vi "Cntrl_Ch_Status_low.vi"(1 "Mode":T1(ring), 2 "Channel names":string[](array[string])) -> (0 "Disabled Chs":string[](array[string]))   [LabVIEW 2020]
uses:
  Sub VIs/ADAM Controls/Channel_State.ctl
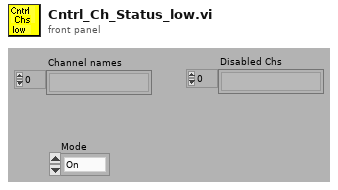
[diagram p1: front panel]
types:
  T1 = enum16{"On", "Off", "Always On", "Always Off", "Delete"}
  T2 = typedef "Channel_State.ctl" = enum16{"On", "Off", "Always On", "Always Off"}
  T3 = typedef "Ch_description_ADAM.ctl" = cluster{"Ch Name":string, "Type":T4, "Function":T5, "Ch State":T2, "Calibration type":T6, "A":dbl, "B":dbl, "C":dbl, "D":dbl, "Comments":string, "Address":T7, "String":string, "Duty":u16}
  T4 = typedef "Module_type_ADAM.ctl" = string
  T5 = typedef "Function_ADAM.ctl" = enum16{"Analogue Input", "Digital Input", "Event counter", "Event rate", "Analogue Output", "Digital Output", "Relay Output"}
  T6 = typedef "Calib_type_ADAM.ctl" = string
  T7 = typedef "Address.ctl" = cluster{"Main":i32, "Ch.":i32, "Sub":i32, "Port Name":string}
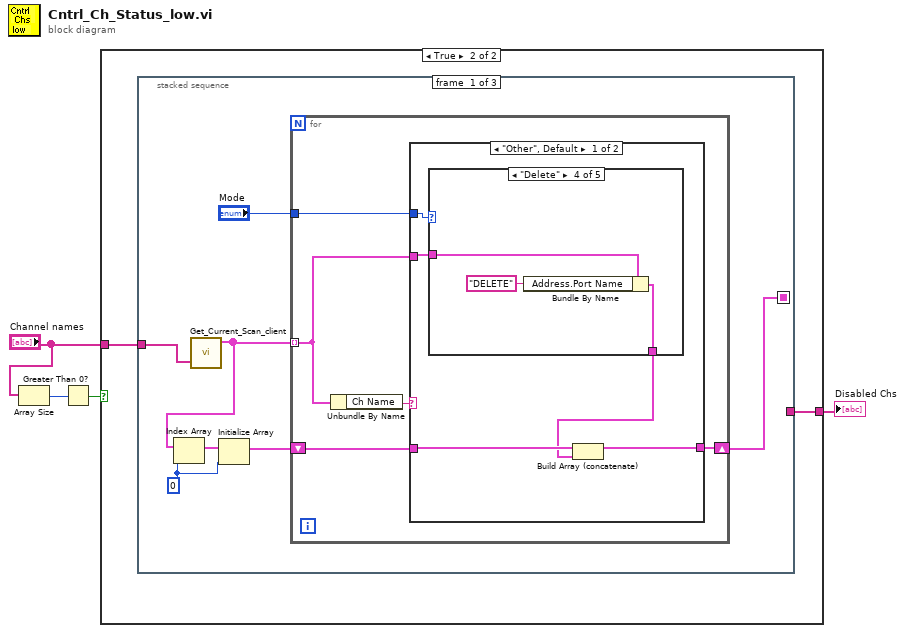
[diagram p0: block diagram]
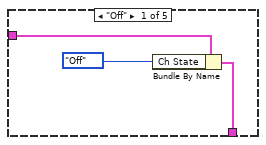
[diagram p3: hidden frame]
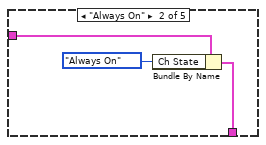
[diagram p4: hidden frame]
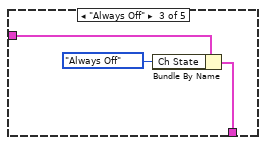
[diagram p5: hidden frame]
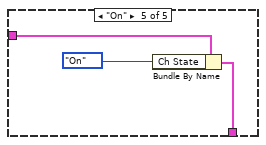
[diagram p6: hidden frame]
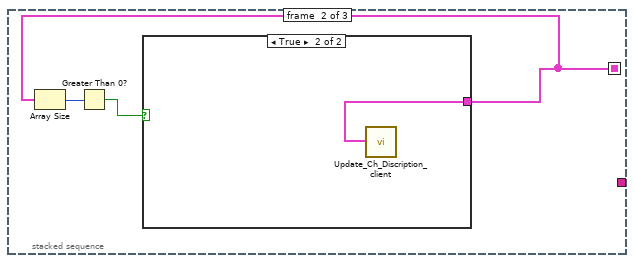
[diagram p8: hidden frame]
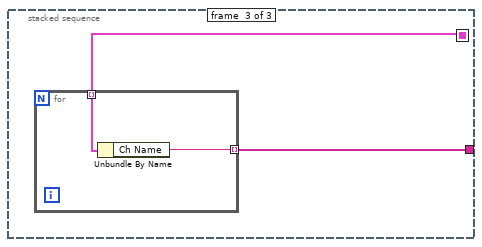
[diagram p10: hidden frame]
diagram:
  n1 = Array Size(array="Channel names") -> (size(s)=w4:i32)
  n2 = Greater Than 0?(x=w4) -> (x > 0?=w2:bool)
  n3 = case shown="True" w2 {
    tunnel: "Channel names" -> [w5 w7]
    tunnel: [w5 w6] -> w1
    frame False {
    }
    frame True {
      n4 = stacked-sequence {
        seq-local: [w9 _ _] -> [_ w41 w46]
        tunnel: w7 -> [w14 _ _]
        tunnel: [_ _ w45] -> w6
        frame #0 {
          w13 = 0 ("Index")
          n5 = call "Get_Current_Scan_client.vi"("multipleChannels"=w14) -> ("Ch Description Array"=w12:T3[])  [unwired: 2 in, 2 out]
          n6 = Index Array(array=w12, index=w13) -> (element=w11:T3)
          n7 = Initialize Array(w11, w13) -> (w10:T3[])
          n8 = for {
            tunnel: w12 -> [w16] mode=indexing
            shift-right: [w18] -> w9
            shift-left: w10 -> [w17]
            tunnel: "Mode" -> [w15]
            n9 = Unbundle By Name(w16) -> ("Ch Name"=w19:string)
            n10 = case shown="\"Other\", Default" w19 {
              tunnel: [w23 w40] -> w18
              tunnel: w17 -> [w24 w40]
              tunnel: w16 -> [w22 _]
              tunnel: w15 -> [w20 _]
              frame "Other", Default {
                n11 = case shown="\"Delete\"" w20 {
                  tunnel: w22 -> [w27 w30 w33 w36 w39]
                  tunnel: [w26 w29 w32 w35 w38] -> w21
                  frame "Off" {
                    n12 = Bundle By Name(cluster=w27, "Ch State"=Channel_State."Off" ("Channel State")) -> (w26:T3)
                  }
                  frame "Always On" {
                    n13 = Bundle By Name(cluster=w30, "Ch State"=Channel_State."Always On" ("Channel State")) -> (w29:T3)
                  }
                  frame "Always Off" {
                    n14 = Bundle By Name(cluster=w33, "Ch State"=Channel_State."Always Off" ("Channel State")) -> (w32:T3)
                  }
                  frame "Delete" {
                    n15 = Bundle By Name(cluster=w36, "Address.Port Name"="DELETE") -> (w35:T3)
                  }
                  frame "On" {
                    n16 = Bundle By Name(cluster=w39, "Ch State"=Channel_State."On" ("Channel State")) -> (w38:T3)
                  }
                }
                n17 = Build Array (concatenate)(w24, w21) -> (w23:T3[])
              }
              frame "No Match" {
              }
            }
          }
        }
        frame #1 {
          n18 = Array Size(array=w41) -> (size(s)=w43:i32)
          n19 = Greater Than 0?(x=w43) -> (x > 0?=w42:bool)
          n20 = case shown="True" w42 {
            tunnel: w41 -> [_ w44]
            frame False {
            }
            frame True {
              n21 = call "Update_Ch_Discription_client.vi"("Channels to update In"=w44) -> ()  [unwired: 1 in]
            }
          }
        }
        frame #2 {
          n22 = for {
            tunnel: w46 -> [w48] mode=indexing
            tunnel: [w47] -> w45 mode=indexing
            n23 = Unbundle By Name(w48) -> ("Ch Name"=w47:string)
          }
        }
      }
    }
  }
  "Disabled Chs" <- w1
